vi "UHR-Fleezers Control (host) - Lorentz v4.vi"() -> ()   [LabVIEW 2014] (continued)
        n116 = local read "Channel 1"() -> (w331:T28)
        n117 = Array To Cluster(array=w333) -> (cluster=w332:T42)
        n118 = local read "Channel 3"() -> (w329:T28)
        n119 = Unbundle(w332) -> ("[0]"=w326:sgl, "[1]"=w325:sgl, "[2]"=w324:sgl, "[3]"=w323:sgl, "[4]"=w322:sgl, "[5]"=w321:sgl, "[6]"=w320:sgl, "[7]"=w319:sgl, "[8]"=w318:sgl, "[9]"=w317:sgl, "[10]"=w316:sgl, "[11]"=w315:sgl, "[12]"=w314:sgl, "[13]"=w313:sgl, "[14]"=w312:sgl)
        n120 = Bundle By Name(cluster=w331, "X Pos (mm)"=w326, "Y Pos (mm)"=w325, "Z Pos (mm)"=w324) -> (w311:T28)
        n121 = Bundle By Name(cluster=w330, "X Pos (mm)"=w323, "Y Pos (mm)"=w322, "Z Pos (mm)"=w321) -> (w310:T28)
        n122 = Bundle By Name(cluster=w328, "X Pos (mm)"=w317, "Y Pos (mm)"=w316, "Z Pos (mm)"=w315) -> (w308:T28)
        n123 = Bundle By Name(cluster=w329, "X Pos (mm)"=w320, "Y Pos (mm)"=w319, "Z Pos (mm)"=w318) -> (w309:T28)
        n124 = Bundle By Name(cluster=w327, "X Pos (mm)"=w314, "Y Pos (mm)"=w313, "Z Pos (mm)"=w312) -> (w307:T28)
        n125 = property on="Channel 2" class="Clust (strict)"("Value"=w310) -> ()  [unwired: 2 in, 2 out]
        n126 = property on="Channel 5" class="Clust (strict)"("Value"=w307) -> ()  [unwired: 2 in, 2 out]
        n127 = property on="Channel 1" class="Clust (strict)"("Value"=w311) -> ()  [unwired: 2 in, 2 out]
        n128 = property on="Channel 3" class="Clust (strict)"("Value"=w309) -> ()  [unwired: 2 in, 2 out]
        n129 = property on="Channel 4" class="Clust (strict)"("Value"=w308) -> ()  [unwired: 2 in, 2 out]
      }
    }
    n130 = Merge Errors(w100, w99, w98) -> (w97:errorcluster)
    n131 = property on="Motor Error Cluster out" class="Clust (strict)"("Val(Sgnl)"=w97) -> ()  [unwired: 2 in, 2 out]
  }
  n132 = disable-structure shown="Disabled" {
    frame Disabled {
      w347 = T34 0 items=["Grayscale (U8)", "Grayscale (I16)", "Grayscale (SGL)", "Complex (CSG)", "RGB (U32)", "HSL (U32)", "RGB (U64)", "Grayscale (U16)"] ("Image Type")
      n133 = call <vilib>:"IMAQdx Open Camera.vi"("Session In"=T43 "cam0") -> ("error out"=w351:errorcluster, "Session Out"=w350:T43)  [unwired: 9 in]
      n134 = call <vilib>:"IMAQdx Configure Grab.vi"("error in"=w351, "Session In"=w350) -> ("error out"=w342:errorcluster, "Session Out"=w349:T43)  [unwired: 8 in]
      n135 = call "IMAQ Create"("Image Name"="untitled", "Image Type"=w347) -> ("New Image"=w353:T1)  [unwired: 3 in, 1 out]
      n136 = while {
        tunnel: w353 -> [w359]
        tunnel: w349 -> [w360]
        tunnel: w342 -> [w358]
        tunnel: [w356] -> w346
        tunnel: [w357] -> w345
        tunnel: [w355] -> w343
        stop <- w354 stop-if-true
        n137 = call <vilib>:"IMAQdx Grab.vi"("error in"=w358, "Image In"=w359, "Session In"=w360) -> ("error out"=w356:errorcluster, "Image Out"=w355:T1, "Session Out"=w357:T43)  [unwired: 5 in, 1 out]
        "Image" <- w355
        n138 = local read "Stop All"() -> (w354:bool)
      }
      n139 = call <vilib>:"IMAQdx Close Camera.vi"("error in"=w346, "Session In"=w345) -> ("error out"=→"error out 4":errorcluster)  [unwired: 9 in]
      n140 = call "IMAQ Dispose"("Image"=w343) -> ()  [unwired: 5 in, 1 out]
    }
    frame Enabled {
    }
  }
  n141 = for {
    tunnel: w14 -> [w363] mode=indexing
    tunnel: w7 -> [w362] mode=indexing
    tunnel: [w361] -> w15 mode=indexing
    n142 = call "TLMotorStopCtrl.vi"("Error In (No Error)"=w362, "Motor Ref"=w363) -> ("Error Out"=w361:errorcluster)  [unwired: 4 in, 1 out]
  }
  n143 = call-poly <vilib>:"Close Input Device.vi"("error in (no error)"=w9, "device ID"=w8) -> ("error out"=w6:errorcluster)  [unwired: 8 in]
  n144 = Merge Errors(w15, w5, w6, w1) -> (→"Motor Error Cluster out":errorcluster)
  n145 = disable-structure shown="Enabled" {
    frame Enabled {
      w390 = FALSE
      # "This Control added by\nRonen to enable direct\nControl of pressure pulse\nlength to enable fine flow\ncontrol"
      # "Start out with all lines set to zero"
      n146 = Format Into String(format string="%s/port0/line5:1, %s/port1/line0:3", "DAQmx Device Name", "DAQmx Device Name") -> (resulting string=w382:string)  [unwired: 2 in, 1 out]
      n147 = Format Into String(format string="%s/ai0", "DAQmx Device Name") -> (resulting string=w380:string)  [unwired: 2 in, 1 out]
      n148 = In Range and Coerce(upper limit=100.0, x="Pulse Duration (0-100 ms)", lower limit=0.0) -> (coerced(x)=w365:dbl)  [unwired: 1 out]
      n149 = Bundle By Name(cluster=T44 {"daqmx_channel"="", "terminal_configuration"=""} ("Pressure Control Config"), "daqmx_channel"=w380, "terminal_configuration"="RSE") -> (w397:T44)
      n150 = To Unsigned Long Integer(number=w365) -> (unsigned 32bit integer=w364:u32)
      n151 = Bundle("Pressure up", "TTL line # Pressure Up"=u8 6, w390, w390) -> (w388:T45)  [unwired: 1 in]
      n152 = Bundle("Pressure down", "TTL line # Pressure Down"=u8 8, w390, w390) -> (w389:T46)  [unwired: 1 in]
      n153 = Bundle("Pressure vacuum", "TTL line # Pressure Vacuum"=u8 7, w390, w390) -> (w387:T47)  [unwired: 1 in]
      n154 = Build Array(w388, w389, w387) -> (w386:T48)
      n155 = call "Initialize.vi"("Pulse duration (ms)"=w364, "TTL Ports"=w382, "TTL in"=refnum<class "TTL.lvclass"> refnum ("TTL.lvclass")) -> ("error out"=w385:errorcluster, "TTL out"=w374:refnum<class "TTL.lvclass">)  [unwired: 7 in]
      n156 = call "Initialize.vi"("TTL Lines"=w386, "error in (no error)"=w385, "TTL"=w374, "Pressure Control Config"=w397, "Pressure Control in"=refnum<class "Pressure Control.lvclass"> refnum ("Pressure Control.lvclass")) -> ("error out"=w402:errorcluster, "Pressure Control out"=w384:refnum<class "Pressure Control.lvclass">)  [unwired: 5 in]
      n157 = call "Get line states.vi"("error in (no error)"=w402, "TTL in"=w374) -> ("error out"=w369:errorcluster, "Current line states"=w370:bool[], "TTL out"=w373:refnum<class "TTL.lvclass">)  [unwired: 7 in]
      n158 = Array Size(array=w370) -> (size(s)=w371:i32)
      n159 = for {
        N: w371 -> [_]
        shift-right: [w408] -> w372
        shift-left: w373 -> [w409]
        shift-right: [w406] -> w403
        shift-left: w369 -> [w407]
        i -> [w405]
        n160 = call "Set line.vi"("error in (no error)"=w407, "Action"=enum16{"Open", "Close", "Toggle"}."Open", "Line number"=w405, "TTL in"=w409) -> ("error out"=w406:errorcluster, "TTL out"=w408:refnum<class "TTL.lvclass">)  [unwired: 6 in]
      }
      n161 = case shown="No Error" w403 {
        selector: w403 -> [_ w463]
        tunnel: w384 -> [w414 _]
        tunnel: w372 -> [w413 _]
        tunnel: [w410 w462] -> w377
        frame No Error {
          n162 = while {
            shift-right: [w422] -> w411
            shift-left: w414 -> [w421]
            shift-right: [w420] -> w412
            shift-left: w413 -> [w419]
            stop <- w417 stop-if-true
            n163 = call "Get pressure.vi"("Pressure Control in"=w421) -> ("Pressure"=→"Pressure":dbl)  [unwired: 7 in, 3 out]
            n164 = event shown="[7] \"Pulse Duration (0-100 ms)\": Value Change" {
              selector: _ -> [_ _ _ _ _ _ _ _]
              dyn-events: _ -> [_ _ _ _ _ _ _ _]
              timeout: 100 -> [_ _ _ _ _ _ _ _]
              tunnel: [w425 w428 w429 w434 w438 w443 w448 w460] -> w422
              tunnel: w421 -> [w425 w428 w430 w435 w439 w444 w449 w461]
              tunnel: [w424 w427 w431 w436 w440 w445 w450 w458] -> w420
              tunnel: w419 -> [w424 w427 w431 w436 w440 w445 w450 w459]
              tunnel: [_ TRUE _ _ _ _ _ _] -> w417
              tunnel: [_ _ w432 w437 w441 w446 w451 w457] -> w416
              event Timeout {
                n165 = event-data() -> ()  [unwired: 1 in, 2 out]
              }
              event "Stop All": Value Change {
                n166 = event-data() -> ()  [unwired: 1 in, 6 out]
              }
              event "Vent pressure": Value Change {
                n167 = event-data() -> ()  [unwired: 1 in, 5 out]
                n168 = call "Vent.vi"("Pressure Control in"=w430) -> ("error out"=w432:errorcluster, "Pressure Control out"=w429:refnum<class "Pressure Control.lvclass">)  [unwired: 9 in]
              }
              event "Vacuum": Value Change {
                n169 = event-data() -> ("NewVal"=w433:bool)  [unwired: 1 in, 4 out]
                n170 = call "Set vacuum.vi"("Vacuum?"=w433, "Pressure Control in"=w435) -> ("error out"=w437:errorcluster, "Pressure Control out"=w434:refnum<class "Pressure Control.lvclass">)  [unwired: 8 in]
              }
              event "Set zero pressure": Value Change {
                n171 = event-data() -> ()  [unwired: 1 in, 5 out]
                n172 = call "Set zero pressure to current pressure.vi"("Pressure Control in"=w439) -> ("error out"=w441:errorcluster, "Pressure Control out"=w438:refnum<class "Pressure Control.lvclass">)  [unwired: 8 in, 1 out]
              }
              event "Pressure Up": Value Change {
                n173 = event-data() -> ()  [unwired: 1 in, 5 out]
                n174 = call "Pressure pulse.vi"("Up or down?"=enum16{"Up", "Down"}."Up", "Pressure Control in"=w444) -> ("error out"=w446:errorcluster, "Pressure Control out"=w443:refnum<class "Pressure Control.lvclass">)  [unwired: 8 in]
              }
              event "Pressure Down": Value Change {
                n175 = event-data() -> ()  [unwired: 1 in, 5 out]
                n176 = call "Pressure pulse.vi"("Up or down?"=enum16{"Up", "Down"}."Down", "Pressure Control in"=w449) -> ("error out"=w451:errorcluster, "Pressure Control out"=w448:refnum<class "Pressure Control.lvclass">)  [unwired: 8 in]
              }
              event "Pulse Duration (0-100 ms)": Value Change {
                # "Event added by Ronen to allow for changes\nin pulse duration as program is running"
                n177 = event-data() -> ()  [unwired: 1 in, 6 out]
                n178 = local read "Pulse Duration (0-100 ms)"() -> (w455:dbl)
                n179 = In Range and Coerce(upper limit=100.0, x=w455, lower limit=0.0) -> (coerced(x)=w453:dbl)  [unwired: 1 out]
                n180 = To Unsigned Long Integer(number=w453) -> (unsigned 32bit integer=w452:u32)
                n181 = call "Change TTL - Ronen.vi"("Pulse Duration (ms)"=w452, "TTL.lvclass"=w459) -> ("error out"=w457:errorcluster, "TTL.lvclass"=w458:refnum<class "TTL.lvclass">)  [unwired: 8 in]
                n182 = call "Update TTL - Ronen.vi"("TTL.lvclass"=w458, "Pressure Control in"=w461) -> ("Pressure Control out"=w460:refnum<class "Pressure Control.lvclass">)  [unwired: 8 in, 1 out]
              }
            }
            n183 = call <vilib>:"Simple Error Handler.vi"("error in (no error)"=w416) -> ()  [unwired: 4 in, 5 out]
          }
          n184 = call "Close.vi"("Pressure Control in"=w411) -> ("error out"=w415:errorcluster)  [unwired: 9 in, 1 out]
          n185 = call "Close.vi"("error in (no error)"=w415, "TTL in"=w412) -> ("error out"=w410:errorcluster)  [unwired: 8 in, 1 out]
        }
        frame Error {
          n186 = call <vilib>:"Simple Error Handler.vi"("error in (no error)"=w463) -> ("error out"=w462:errorcluster)  [unwired: 4 in, 4 out]
        }
      }
      n187 = property on="DAQmx Device Name" class="DAQmxName"("Visible"=FALSE) -> ()  [unwired: 2 in, 2 out]
      n188 = call <vilib>:"Clear Errors.vi"("error in (no error)"=w377) -> ("error out"=w375:errorcluster)  [unwired: 5 in, 1 out]
      n189 = property on="DAQmx Device Name" class="DAQmxName"(error in=w375, "Visible"=TRUE) -> ()  [unwired: 1 in, 2 out]
    }
    frame Disabled {
    }
  }
  n190 = disable-structure shown="Disabled" {
    disable-tunnel: [w495 _] -> w76
    disable-tunnel: [w492 _] -> w65
    disable-tunnel: [w491 _] -> w64
    disable-tunnel: [w486 _] -> w60
    disable-tunnel: [w485 _] -> w59
    disable-tunnel: [w484 _] -> w58
    disable-tunnel: [w483 _] -> w57
    disable-tunnel: [w480 _] -> w49
    disable-tunnel: [w475 _] -> w30
    disable-tunnel: [w468 _] -> w29
    disable-tunnel: [w465 _] -> w28
    frame Disabled {
      w467 = u16 20 items=["1.0"=10, "1.5"=15, "2.0"=20] ("stop bits (10: 1 bit)")
      w478 = u16 20 items=["1.0"=10, "1.5"=15, "2.0"=20] ("stop bits (10: 1 bit)")
      w481 = u16 10 items=["1.0"=10, "1.5"=15, "2.0"=20] ("stop bits (10: 1 bit)")
      w487 = u16 20 items=["1.0"=10, "1.5"=15, "2.0"=20] ("stop bits (10: 1 bit)")
      w489 = u16 20 items=["1.0"=10, "1.5"=15, "2.0"=20] ("stop bits (10: 1 bit)")
      w493 = u16 20 items=["1.0"=10, "1.5"=15, "2.0"=20] ("stop bits (10: 1 bit)")
      # "Bottom 1 Harvard"
      # "Top 3 Harvard"
      # "Center Harvard"
      n191 = call-poly "VISA Configure Serial Port"("VISA resource name"=refnum<visa-resource-name> "COM2", "baud rate (9600)"=u32 9600, "stop bits (10: 1 bit)"=w478) -> ("VISA resource name out"=w468:refnum<visa-resource-name>, "error out"=→"Preamp Error Out":errorcluster)  [unwired: 4 in, 7 out]
      n192 = call-poly "VISA Configure Serial Port"("VISA resource name"=refnum<visa-resource-name> "COM2", "baud rate (9600)"=u32 9600, "stop bits (10: 1 bit)"=w467) -> ("VISA resource name out"=w465:refnum<visa-resource-name>)  [unwired: 4 in, 8 out]
      n193 = call-poly "VISA Configure Serial Port"("VISA resource name"=refnum<visa-resource-name> "COM7", "baud rate (9600)"=u32 115200, "stop bits (10: 1 bit)"=w481) -> ("VISA resource name out"=w480:refnum<visa-resource-name>, "error out"=w479:errorcluster)  [unwired: 4 in, 7 out]
      n194 = call-poly "VISA Configure Serial Port"("VISA resource name"=refnum<visa-resource-name> "COM5", "baud rate (9600)"=u32 115200, "stop bits (10: 1 bit)"=w487) -> ("VISA resource name out"=w484:refnum<visa-resource-name>, "error out"=w483:errorcluster)  [unwired: 4 in, 7 out]
      n195 = call-poly "VISA Configure Serial Port"("VISA resource name"=refnum<visa-resource-name> "COM4", "baud rate (9600)"=u32 115200, "stop bits (10: 1 bit)"=w489) -> ("VISA resource name out"=w486:refnum<visa-resource-name>, "error out"=w485:errorcluster)  [unwired: 4 in, 7 out]
      n196 = call-poly "VISA Configure Serial Port"("VISA resource name"=refnum<visa-resource-name> "COM6", "baud rate (9600)"=u32 115200, "stop bits (10: 1 bit)"=w493) -> ("VISA resource name out"=w491:refnum<visa-resource-name>, "error out"=w492:errorcluster)  [unwired: 4 in, 7 out]
      n197 = call-poly "VISA Configure Serial Port"("VISA resource name"=refnum<visa-resource-name> "COM1") -> ("VISA resource name out"=w475:refnum<visa-resource-name>, "error out"=w495:errorcluster)  [unwired: 5 in, 8 out]
      "Stage Control Serial Error" <- w495
      n198 = local write "Blue Error Out"(w479) -> ()
    }
    frame Enabled {
    }
  }
  n199 = call "IMAQ Create"("Image Name"="APD 1 Image", "Image Type"=w53) -> ("New Image"=w70:T1)  [unwired: 3 in, 1 out]
  n200 = call "IMAQ Create"("Image Name"="APD 2 Image", "Image Type"=w53) -> ("New Image"=w69:T1)  [unwired: 3 in, 1 out]
  n201 = call "IMAQ Create"("Image Name"="APD 3 Image", "Image Type"=w53) -> ("New Image"=w52:T1)  [unwired: 3 in, 1 out]
  n202 = call "IMAQ Create"("Image Name"="Det. X Image", "Image Type"=w53) -> ("New Image"=w68:T1)  [unwired: 3 in, 1 out]
  n203 = call "IMAQ Create"("Image Name"="Det. Y Image", "Image Type"=w53) -> ("New Image"=w67:T1)  [unwired: 3 in, 1 out]
  n204 = Bundle("New Image"=w70, "New Image"=w69, "New Image"=w52, "New Image"=w68, "New Image"=w67) -> (w66:T49)  [unwired: 1 in]
  n205 = xnode "Open FPGA VI Reference"("resource name"=T33 "RIO0") -> ("FPGA VI Reference Out"=w47:T50, "error out"=w46:errorcluster)  [unwired: 1 in]
  n206 = xnode "Invoke Method"("FPGA VI Reference In"=w47, "error in"=w46) -> ("FPGA VI Reference Out"=w27:T50, "error out"=→"FPGA error out":errorcluster)
  n207 = Subtract(x=w25, y="Maximum Delta\n(MHz)") -> (x-y=w23:dbl)
  n208 = Bundle By Name(cluster=T24 {"Minimum"=60.0, "Maximum"=90.0, "Increment"=1.0} ("Min Max Inc"), "Minimum"=w23, "Maximum"=w25) -> (w22:T24)
  n209 = node-c288() -> (w73:T35)  [unwired: 4 in]
  n210 = timed-loop "Run Scripts, including: stage motion" {
    tunnel: w76 -> [w506]
    tunnel: w30 -> [w507]
    tunnel: [w507] -> w75
    tunnel: [w506] -> w74
    timing: w73 -> [_]
    timing-out: [_] -> w72
    tunnel: w64 -> [w505]
    tunnel: w65 -> [w504]
    tunnel: w60 -> [w501]
    tunnel: w59 -> [w500]
    tunnel: w58 -> [w502]
    tunnel: w57 -> [w503]
    tunnel: w49 -> [w499]
    tunnel: w42 -> [w498]
    tunnel: w29 -> [w497]
    tunnel: w28 -> [w496]
    stop <- w508 stop-if-true
    n211 = node-c288() -> ()  [unwired: 1 in, 1 out]
    n212 = event shown="[17] \"Got Bead 1\": Value Change" {
      selector: _ -> [_ _ _ _ _ _ _ _ _ _ _ _ _ _ _ _ _ _ _ _ _ _ _ _ _ _ _ _]
      dyn-events: _ -> [_ _ _ _ _ _ _ _ _ _ _ _ _ _ _ _ _ _ _ _ _ _ _ _ _ _ _ _]
      timeout: _ -> [_ _ _ _ _ _ _ _ _ _ _ _ _ _ _ _ _ _ _ _ _ _ _ _ _ _ _ _]
      tunnel: ["Set Position" "Move to Position" _ _ _ _ _ _ "Read Harvard" _ _ _ _ _ _ _ _ "Got Bead 1" "Force FB Data\nScript" _ "Got Bead 2" _ "Take Stepping Data" _ "Take Detection Laser\nImage" _ _ _] -> _
      tunnel: [_ _ _ _ _ _ _ _ _ _ _ _ _ _ _ _ _ _ _ _ _ _ _ _ _ _ w1435 _] -> w508
      tunnel: w506 -> [w527 w535 w548 w578 _ _ _ _ _ w715 w749 w775 w807 w896 w925 w1057 w1084 _ w1126 _ _ _ _ _ _ _ _ _]
      tunnel: w507 -> [w528 w536 w549 w579 _ _ _ _ _ w716 w750 w776 w808 w897 w926 w1058 w1085 _ w1127 _ _ _ _ _ _ _ _ _]
      tunnel: w505 -> [_ _ _ _ _ _ _ _ w700 _ _ _ _ _ _ _ _ _ _ _ _ _ _ _ _ _ _ _]
      tunnel: w504 -> [_ _ _ _ _ _ _ _ w699 _ _ _ _ _ _ _ _ _ _ _ _ _ _ _ _ _ _ _]
      tunnel: w503 -> [_ _ _ _ _ _ _ _ _ _ _ _ _ _ _ _ _ _ _ _ _ _ _ _ _ _ _ _]
      tunnel: w502 -> [_ _ _ _ _ _ _ _ _ _ _ _ _ _ _ _ _ _ _ _ _ _ _ _ _ _ _ _]
      tunnel: w501 -> [_ _ _ _ _ _ _ _ _ _ _ _ _ _ _ _ _ _ _ _ _ _ _ _ _ _ _ _]
      tunnel: w500 -> [_ _ _ _ _ _ _ _ _ _ _ _ _ _ _ _ _ _ _ _ _ _ _ _ _ _ _ _]
      tunnel: w499 -> [_ _ _ _ w606 w613 w641 w660 _ _ _ _ _ _ _ _ _ _ _ _ _ _ _ _ _ _ w1434 _]
      tunnel: w498 -> [_ _ _ _ _ _ _ _ _ _ _ _ _ _ _ _ _ _ _ _ _ _ _ _ _ w1301 _ _]
      tunnel: w497 -> [_ _ _ _ _ _ _ _ _ _ _ _ _ _ _ _ _ _ _ _ _ _ _ _ _ _ _ w1445]
      tunnel: w496 -> [_ _ _ _ _ _ _ _ _ _ _ _ _ _ _ _ _ _ _ _ _ _ _ _ _ _ _ w1440]
      tunnel: [_ _ _ _ _ _ _ _ _ _ _ _ _ _ _ _ _ _ _ _ _ "Get New Beads" _ _ _ _ _ _] -> _
      event "Set Position", "Set Position 2", "Set Position 3", "Set Position 4", "Set Position 5", "Set Position 1", "Set Position 6": Value Change {
        n213 = event-data() -> ()  [unwired: 1 in, 5 out]
        n214 = Build Array("Set Position 1", "Set Position 2", "Set Position 3", "Set Position 4", "Set Position 5", "Set Position 6") -> (w526:bool[])
        n215 = Boolean Array To Number(Boolean array=w526) -> (number=w525:u32)
        n216 = Logarithm Base 2(1:w525) -> (0:w517:dbl)
        n217 = call "Read Stage Position.vi"("error in"=w527, "VISA resource name in"=w528) -> ("Current Position"=w532:cluster{dbl, dbl, dbl}, "error out"=w531:errorcluster)  [unwired: 2 out]
        n218 = Decrement(x="Position") -> (x-1=w515:dbl)
        n219 = Greater Or Equal?(x=w517, y=0.0) -> (x >= y?=w518:bool)
        n220 = Cluster To Array(cluster=w532) -> (array=w529:dbl[])
        n221 = local write "Stage Control Serial Error"(w531) -> ()
        n222 = Select(t=w517, s=w518, f=w515) -> (s? t:f=w514:dbl)
        n223 = Increment(x=w514) -> (x+1=w513:dbl)
        n224 = Build Array (concatenate)(w513, w529) -> (w512:dbl[])
        n225 = Replace Array Subset(array="Saved Stage Positions", new element=w512, index (row)=w514) -> (w530:dbl[][])  [unwired: 1 in]
        n226 = local write "Saved Stage Positions"(w530) -> ()
      }
      event "Move to Position": Value Change {
        n227 = event-data() -> ()  [unwired: 1 in, 5 out]
        n228 = flat-sequence {
          tunnel: w536 -> [w540]
          tunnel: w535 -> [w539]
          frame #0 {
            n229 = local read "Saved Stage Positions"() -> (w542:dbl[][])
            n230 = local read "Position"() -> (w541:dbl)
            n231 = local write "Stage Moving"(TRUE ("Stage Moving")) -> ()
            n232 = call "move to saved stage position.vi"("error in"=w539, "Stage VISA resource name in"=w540, "Position"=w541, "Saved Stage Positions"=w542) -> ("error out"=w538:errorcluster)  [unwired: 1 out]
            n233 = local write "Stage Control Serial Error"(w538) -> ()
          }
          frame #1 {
            n234 = call <vilib>:"Beep.vi"() -> ()  [unwired: 3 in, 9 out]
            n235 = local write "Stage Moving"(FALSE ("Stage Moving")) -> ()
          }
        }
      }
      event "Move Cap. 1 (DNA Bottom)": Value Change {
        n236 = event-data() -> ()  [unwired: 1 in, 5 out]
        n237 = local write "Move Cap. 1 (DNA Bottom)"(FALSE ("Move Cap. 1 (DNA Right)")) -> ()
        n238 = flat-sequence {
          tunnel: w548 -> [w551]
          tunnel: w549 -> [w552]
          tunnel: [w552] -> w546
          tunnel: [w551] -> w545
          tunnel: w546 -> [w554]
          tunnel: w545 -> [w553]
          frame #0 {
            n239 = property on="Sample Channel\nFlow" class="Bool (strict)"("Val(Sgnl)"="Cap 1 Samp Flow ON") -> ()  [unwired: 2 in, 2 out]
          }
          frame #1 {
            n240 = local read "Saved Stage Positions"() -> (w564:dbl[][])
            n241 = local write "Stage Moving"(TRUE ("Stage Moving")) -> ()
            n242 = Array Subset(array=w564, index (row)=0 ("index"), length (row)=1 ("length"), index (col)=1 ("index"), length (col)=3 ("length")) -> (w561:dbl[][])
            n243 = Reshape Array(w561, 3 ("dimension size")) -> (w559:dbl[])
            n244 = Array To Cluster(array=w559) -> (cluster=w558:cluster{"[0]":dbl, "[1]":dbl, "[2]":dbl})
            n245 = call "Set Stage Position.vi"("Position"=w558, "error in"=w553, "VISA resource name in"=w554) -> ("error out"=w557:errorcluster)  [unwired: 2 out]
            n246 = local write "Stage Control Serial Error"(w557) -> ()
          }
          frame #2 {
            n247 = local write "Stage Moving"(FALSE ("Stage Moving")) -> ()
            n248 = case shown="True" "Cap 1 Flow ON" {
              frame False {
              }
              frame True {
                n249 = property on="Inject Pump 1" class="Bool (strict)"("Val(Sgnl)"=TRUE ("Value (Signaling)")) -> ()  [unwired: 2 in, 2 out]
              }
            }
            n250 = call <vilib>:"Beep.vi"() -> ()  [unwired: 3 in, 9 out]
          }
          frame #3 {
            n251 = property on="Sample Channel\nFlow" class="Bool (strict)"("Val(Sgnl)"=FALSE ("Value (Signaling)")) -> ()  [unwired: 2 in, 2 out]
            n252 = local read "Cap. 2 BD T1?\n(ADig T1, DNA T2)"() -> (w571:bool)
            n253 = case shown="True" w571 {
              tunnel: "Cap 1 T ON" -> [w573 w574]
              frame False {
                n254 = property on="Trap 1 (ON/OFF)" class="Bool (strict)"("Val(Sgnl)"=w573) -> ()  [unwired: 2 in, 2 out]
              }
              frame True {
                n255 = property on="Trap 2 (ON/OFF)" class="Bool (strict)"("Val(Sgnl)"=w574) -> ()  [unwired: 2 in, 2 out]
              }
            }
            n256 = property on="Got Bead 2" class="Bool"("Key Focus"=TRUE) -> ()  [unwired: 2 in, 2 out]
          }
        }
      }
      event "Move Cap. 2 (ADig Top)": Value Change {
        n257 = event-data() -> ()  [unwired: 1 in, 5 out]
        n258 = local write "Move Cap. 2 (ADig Top)"(FALSE ("Move Cap. 2 (ADig Left)")) -> ()
        n259 = flat-sequence {
          tunnel: w578 -> [w581]
          tunnel: w579 -> [w582]
          tunnel: [w582] -> w576
          tunnel: [w581] -> w575
          tunnel: w576 -> [w585]
          tunnel: w575 -> [w584]
          frame #0 {
            n260 = property on="Sample Channel\nFlow" class="Bool (strict)"("Val(Sgnl)"="Cap 2 Samp Flow ON") -> ()  [unwired: 2 in, 2 out]
          }
          frame #1 {
            w583 = FALSE ("Value (Signaling)")
            n261 = local read "Saved Stage Positions"() -> (w595:dbl[][])
            n262 = local write "Stage Moving"(TRUE ("Stage Moving")) -> ()
            n263 = Array Subset(array=w595, index (row)=1 ("index"), length (row)=1 ("length"), index (col)=1 ("index"), length (col)=3 ("length")) -> (w592:dbl[][])
            n264 = Reshape Array(w592, 3 ("dimension size")) -> (w590:dbl[])
            n265 = property on="Trap 1 (ON/OFF)" class="Bool (strict)"("Val(Sgnl)"=w583) -> ()  [unwired: 2 in, 2 out]
            n266 = property on="Trap 1 (ON/OFF)" class="Bool (strict)"("Val(Sgnl)"=w583) -> ()  [unwired: 2 in, 2 out]
            n267 = Array To Cluster(array=w590) -> (cluster=w589:cluster{"[0]":dbl, "[1]":dbl, "[2]":dbl})
            n268 = call "Set Stage Position.vi"("Position"=w589, "error in"=w584, "VISA resource name in"=w585) -> ("error out"=w588:errorcluster)  [unwired: 2 out]
            n269 = local write "Stage Control Serial Error"(w588) -> ()
          }
          frame #2 {
            n270 = local write "Stage Moving"(FALSE ("Stage Moving")) -> ()
            n271 = call <vilib>:"Beep.vi"() -> ()  [unwired: 3 in, 9 out]
            n272 = case shown="True" "Cap 2 Flow ON" {
              frame False {
              }
              frame True {
                n273 = property on="Inject Pump 3" class="Bool (strict)"("Val(Sgnl)"=TRUE ("Value (Signaling)")) -> ()  [unwired: 2 in, 2 out]
              }
            }
          }
          frame #3 {
            n274 = property on="Sample Channel\nFlow" class="Bool (strict)"("Val(Sgnl)"=FALSE ("Value (Signaling)")) -> ()  [unwired: 2 in, 2 out]
            n275 = case shown="False" "Cap. 2 BD T1?\n(ADig T1, DNA T2)" {
              tunnel: "Cap 2 T ON" -> [w604 w605]
              frame False {
                n276 = property on="Trap 2 (ON/OFF)" class="Bool (strict)"("Val(Sgnl)"=w604) -> ()  [unwired: 2 in, 2 out]
              }
              frame True {
                n277 = property on="Trap 1 (ON/OFF)" class="Bool (strict)"("Val(Sgnl)"=w605) -> ()  [unwired: 2 in, 2 out]
              }
            }
            n278 = property on="Got Bead 1" class="Bool"("Key Focus"=TRUE) -> ()  [unwired: 2 in, 2 out]
          }
        }
      }
      event "Send string\nto Blue Laser": Value Change {
        n279 = event-data() -> ()  [unwired: 1 in, 5 out]
        n280 = flat-sequence {
          tunnel: w606 -> [w607]
          frame #0 {
            n281 = call "serial write macro.vi"("String"="command string", "Delay (ms)"="Delay (ms)", "VISA resource name"=w607) -> ("read buffer"=→"read blue buffer":string, "error out"=→"Blue Error Out":errorcluster)  [unwired: 1 out]
            "command string sent" <- "command string"
          }
          frame #1 {
            n282 = local write "Send string\nto Blue Laser"(FALSE ("Send string")) -> ()
          }
        }
      }
      event "Get Blue Laser State": Value Change {
        n283 = event-data() -> ()  [unwired: 1 in, 5 out]
        n284 = local read "Delay (ms)"() -> (w614:i32)
        n285 = flat-sequence {
          tunnel: w614 -> [w622]
          tunnel: w613 -> [w625]
          tunnel: [w623] -> w618
          tunnel: [w622] -> w617
          tunnel: [w632] -> w616
          tunnel: [w629] -> w615
          tunnel: w618 -> [w630]
          tunnel: w617 -> [w629]
          tunnel: w616 -> [w638]
          tunnel: w615 -> [w636]
          frame #0 {
            w620 = "l?"
            n286 = local write "command string sent"(w620) -> ()
            n287 = call "serial write macro.vi"("String"=w620, "Delay (ms)"=w622, "VISA resource name"=w625) -> ("read buffer"=w621:string, "VISA resource name out"=w623:refnum<visa-resource-name>)  [unwired: 1 out]
            n288 = Decimal String To Number(string=w621) -> (number=w624:i32)  [unwired: 2 in, 1 out]
            n289 = Not Equal To 0?(x=w624) -> (x != 0?=→"Laser On":bool)
            n290 = local write "read blue buffer"(w621) -> ()
          }
          frame #1 {
            w627 = "games?" ("String")
            n291 = local write "command string sent"(w627) -> ()
            n292 = call "serial write macro.vi"("String"=w627, "Delay (ms)"=w629, "VISA resource name"=w630) -> ("read buffer"=w628:string, "VISA resource name out"=w632:refnum<visa-resource-name>)  [unwired: 1 out]
            n293 = Decimal String To Number(string=w628) -> (number=w631:i32)  [unwired: 2 in, 1 out]
            n294 = local write "read blue buffer"(w628) -> ()
            n295 = Not Equal To 0?(x=w631) -> (x != 0?=→"Analog Modulation":bool)
          }
          frame #2 {
            w634 = "gdmes?" ("String")
            n296 = local write "command string sent"(w634) -> ()
            n297 = call "serial write macro.vi"("String"=w634, "Delay (ms)"=w636, "VISA resource name"=w638) -> ("read buffer"=w635:string)  [unwired: 2 out]
            n298 = Decimal String To Number(string=w635) -> (number=w637:i32)  [unwired: 2 in, 1 out]
            n299 = Not Equal To 0?(x=w637) -> (x != 0?=→"Digital Modulation":bool)
            n300 = local write "read blue buffer"(w635) -> ()
          }
          frame #3 {
            n301 = local write "Get Blue Laser State"(FALSE) -> ()
          }
        }
      }
      event "Blue Laser Power (mW)\n(Constant Power Mode)", "Blue Laser Modulation\nPower (mW)": Value Change {
        n302 = event-data() -> ()  [unwired: 1 in, 5 out]
        n303 = flat-sequence {
          tunnel: w641 -> [w647]
          tunnel: [w645] -> w640
          tunnel: w640 -> [w654]
          frame #0 {
            n304 = local read "Delay (ms)"() -> (w646:i32)
            n305 = Concatenate Strings("slmp " ("string"), "Blue Laser Modulation\nPower (mW)") -> (w642:string)
            n306 = call "serial write macro.vi"("String"=w642, "Delay (ms)"=w646, "VISA resource name"=w647) -> ("read buffer"=w643:string, "error out"=w644:errorcluster, "VISA resource name out"=w645:refnum<visa-resource-name>)
            n307 = local write "command string sent"(w642) -> ()
            n308 = local write "read blue buffer"(w643) -> ()
            n309 = local write "Blue Error Out"(w644) -> ()
          }
          frame #1 {
            n310 = local read "Delay (ms)"() -> (w653:i32)
            n311 = Concatenate Strings("p " ("string"), "Blue Laser Power (mW)\n(Constant Power Mode)") -> (w650:string)
            n312 = call "serial write macro.vi"("String"=w650, "Delay (ms)"=w653, "VISA resource name"=w654) -> ("read buffer"=w651:string, "error out"=w652:errorcluster)  [unwired: 1 out]
            n313 = local write "command string sent"(w650) -> ()
            n314 = local write "read blue buffer"(w651) -> ()
            n315 = local write "Blue Error Out"(w652) -> ()
          }
        }
      }
      event "Laser interlacing mode", "Blue Laser Modulation Mode", "Blue Laser ON": Value Change {
        n316 = event-data() -> ()  [unwired: 1 in, 5 out]
        n317 = flat-sequence {
          tunnel: w660 -> [w665]
          tunnel: [w664] -> w657
          tunnel: [w670] -> w659
          tunnel: w657 -> [w673]
          tunnel: w659 -> [w685]
          tunnel: [w679] -> w658
          tunnel: w658 -> [w692]
          frame #0 {
            n318 = local read "Blue Laser ON"() -> (w662:bool)
            n319 = local read "Delay (ms)"() -> (w663:i32)
            n320 = case shown="False" w662 {
              tunnel: ["l0" "l1"] -> w661
              frame False {
              }
              frame True {
              }
            }
            n321 = call "serial write macro.vi"("String"=w661, "Delay (ms)"=w663, "VISA resource name"=w665) -> ("error out"=w666:errorcluster, "VISA resource name out"=w664:refnum<visa-resource-name>)  [unwired: 1 out]
            n322 = local write "Blue Error Out"(w666) -> ()
          }
          frame #1 {
            n323 = local read "Laser interlacing mode"() -> (w675:enum32{"Laser ON", "Laser OFF", "Interlace"})
            n324 = case shown="\"Laser ON\"" w675 {
              tunnel: ["cp" "em" "l0"] -> w669
              frame "Laser ON" {
              }
              frame "Interlace" {
              }
              frame "Laser OFF", Default {
              }
            }
            n325 = local read "Delay (ms)"() -> (w674:i32)
            n326 = call "serial write macro.vi"("String"=w669, "Delay (ms)"=w674, "VISA resource name"=w673) -> ("read buffer"=w671:string, "error out"=w672:errorcluster, "VISA resource name out"=w670:refnum<visa-resource-name>)
            n327 = local write "command string sent"(w669) -> ()
            n328 = local write "read blue buffer"(w671) -> ()
            n329 = local write "Blue Error Out"(w672) -> ()
          }
          frame #2 {
            n330 = case shown="\"Analog Modulation\"" "Blue Laser Modulation Mode" {
              tunnel: ["sdmes 0" "sdmes 1" "sdmes 1"] -> w680
              frame "Analog Modulation" {
              }
              frame "Digital + Analog Modulation" {
              }
              frame "Digital Modulation", Default {
              }
            }
            n331 = local read "Delay (ms)"() -> (w683:i32)
            n332 = call "serial write macro.vi"("String"=w680, "Delay (ms)"=w683, "VISA resource name"=w685) -> ("read buffer"=w681:string, "error out"=w682:errorcluster, "VISA resource name out"=w679:refnum<visa-resource-name>)
            n333 = local write "command string sent"(w680) -> ()
            n334 = local write "read blue buffer"(w681) -> ()
            n335 = local write "Blue Error Out"(w682) -> ()
          }
          frame #3 {
            n336 = local read "Blue Laser Modulation Mode"() -> (w694:string)
            n337 = case shown="\"Digital Modulation\", Default" w694 {
              tunnel: ["sames 1" "sames 1" "sames 0"] -> w690
              frame "Analog Modulation" {
              }
              frame "Digital + Analog Modulation" {
              }
              frame "Digital Modulation", Default {
              }
            }
            n338 = local read "Delay (ms)"() -> (w693:i32)
            n339 = local write "command string sent"(w690) -> ()
            n340 = call "serial write macro.vi"("String"=w690, "Delay (ms)"=w693, "VISA resource name"=w692) -> ("read buffer"=w691:string, "error out"=w689:errorcluster)  [unwired: 1 out]
            n341 = local write "read blue buffer"(w691) -> ()
            n342 = local write "Blue Error Out"(w689) -> ()
          }
        }
      }
      event "Read Harvard": Value Change {
        n343 = event-data() -> ()  [unwired: 1 in, 5 out]
        n344 = Concatenate Strings("write buffer", "\r") -> (w702:string)
        n345 = VISA Write(VISA resource name=w700, write buffer=w702, error in (no error)=w699) -> (VISA resource name out=w711:refnum<visa-resource-name>, error out=w710:errorcluster)  [unwired: 1 out]
        n346 = stacked-sequence {
          tunnel: [w714] -> w709
          tunnel: w711 -> [w714]
          tunnel: w710 -> [w713]
          tunnel: [w713] -> w704
          frame #0 {
            n347 = Wait (ms)(milliseconds to wait=50) -> ()  [unwired: 1 out]
          }
        }
        n348 = property class="Instr"(reference=w709, error in=w704) -> (reference out=w708:refnum<visa-resource-name>, error out=w706:errorcluster, "Serial Settings:Number of Bytes at Serial Port"=w707:u32)
        "Serial Settings:Number of Bytes at Serial Port" <- w707
        n349 = VISA Read(VISA resource name=w708, byte count=w707, error in (no error)=w706) -> (read buffer=w705:string)  [unwired: 3 out]
        "read buffer" <- w705
        n350 = Fract/Exp String To Number(string=w705) -> ()  [unwired: 5 out]
      }
      event "+z", "-z": Value Change {
        n351 = event-data() -> ()  [unwired: 1 in, 5 out]
        n352 = flat-sequence {
          tunnel: w715 -> [w737]
          tunnel: w716 -> [w717]
          frame #0 {
            n353 = call "Read Stage Position.vi"("error in"=w737, "VISA resource name in"=w717) -> ("Current Position"=w722:cluster{dbl, dbl, dbl}, "error out"=w735:errorcluster, "VISA resource name out"=w736:refnum<visa-resource-name>)  [unwired: 1 out]
            n354 = local read "Saved Stage Positions"() -> (w746:dbl[][])
            n355 = Divide(x="z nudge increment (um)", y=1000.0) -> (x/y=w734:dbl)
            n356 = Boolean To (0,1)(Boolean="+z") -> (0, 1=w726:i16)
            n357 = Boolean To (0,1)(Boolean="-z") -> (0, 1=w727:i16)
            n358 = Array Subset(array=w746, index (row)=1 ("index"), length (row)=1 ("length"), index (col)=1 ("index"), length (col)=3 ("length")) -> (w743:dbl[][])
            n359 = Multiply(x=w726, y=w734) -> (x*y=w730:dbl)
            n360 = Multiply(x=w727, y=w734) -> (x*y=w728:dbl)
            n361 = Unbundle(w722) -> (w720:dbl, w719:dbl, w723:dbl)
            n362 = Negate(x=w728) -> (-x=w729:dbl)
            n363 = Reshape Array(w743, 3 ("dimension size")) -> (w741:dbl[])
            n364 = Add(x=w730, y=w729) -> (x+y=w731:dbl)
            n365 = Array To Cluster(array=w741) -> ()  [unwired: 1 out]
            n366 = Add(x=w731, y=w723) -> (x+y=w721:dbl)
            n367 = Bundle(cluster=w722, w720, w719, w721) -> (w718:cluster{dbl, dbl, dbl})
            n368 = call "Set Stage Position.vi"("Position"=w718, "error in"=w735, "VISA resource name in"=w736) -> ("error out"=w740:errorcluster)  [unwired: 2 out]
            n369 = local write "Stage Moving"(TRUE ("Stage Moving")) -> ()
            n370 = local write "Stage Control Serial Error"(w740) -> ()
          }
          frame #1 {
            n371 = local write "Stage Moving"(FALSE ("Stage Moving")) -> ()
          }
        }
      }
      event "-y", "+y": Value Change {
        n372 = event-data() -> ()  [unwired: 1 in, 5 out]
        n373 = flat-sequence {
          tunnel: w749 -> [w773]
          tunnel: w750 -> [w756]
          frame #0 {
            n374 = call "Read Stage Position.vi"("error in"=w773, "VISA resource name in"=w756) -> ("Current Position"=w759:cluster{dbl, dbl, dbl}, "error out"=w771:errorcluster, "VISA resource name out"=w772:refnum<visa-resource-name>)  [unwired: 1 out]
            n375 = Divide(x="y nudge increment (um", y=1000.0) -> (x/y=w770:dbl)
            n376 = Boolean To (0,1)(Boolean="+y") -> (0, 1=w762:i16)
            n377 = Boolean To (0,1)(Boolean="-y") -> (0, 1=w763:i16)
            n378 = Multiply(x=w762, y=w770) -> (x*y=w766:dbl)
            n379 = Multiply(x=w763, y=w770) -> (x*y=w764:dbl)
            n380 = Unbundle(w759) -> (w758:dbl, w753:dbl, w755:dbl)
            n381 = Negate(x=w764) -> (-x=w765:dbl)
            n382 = Add(x=w766, y=w765) -> (x+y=w767:dbl)
            n383 = Add(x=w767, y=w753) -> (x+y=w754:dbl)
            n384 = Bundle(cluster=w759, w758, w754, w755) -> (w757:cluster{dbl, dbl, dbl})
            n385 = call "Set Stage Position.vi"("Position"=w757, "error in"=w771, "VISA resource name in"=w772) -> ("error out"=w752:errorcluster)  [unwired: 2 out]
            n386 = local write "Stage Control Serial Error"(w752) -> ()
            n387 = local write "Stage Moving"(TRUE ("Stage Moving")) -> ()
          }
          frame #1 {
            n388 = local write "Stage Moving"(FALSE ("Stage Moving")) -> ()
          }
        }
      }
      event "-x", "+x": Value Change {
        n389 = event-data() -> ()  [unwired: 1 in, 5 out]
        n390 = flat-sequence {
          tunnel: w775 -> [w799]
          tunnel: w776 -> [w783]
          frame #0 {
            n391 = call "Read Stage Position.vi"("error in"=w799, "VISA resource name in"=w783) -> ("Current Position"=w785:cluster{dbl, dbl, dbl}, "error out"=w797:errorcluster, "VISA resource name out"=w798:refnum<visa-resource-name>)  [unwired: 1 out]
            n392 = Divide(x="x nudge increment (um)", y=1000.0) -> (x/y=w796:dbl)
            n393 = Boolean To (0,1)(Boolean="+x") -> (0, 1=w788:i16)
            n394 = Boolean To (0,1)(Boolean="-x") -> (0, 1=w789:i16)
            n395 = Multiply(x=w788, y=w796) -> (x*y=w792:dbl)
            n396 = Multiply(x=w789, y=w796) -> (x*y=w790:dbl)
            n397 = Unbundle(w785) -> (w777:dbl, w779:dbl, w782:dbl)
            n398 = Negate(x=w790) -> (-x=w791:dbl)
            n399 = Add(x=w792, y=w791) -> (x+y=w793:dbl)
            n400 = Add(x=w793, y=w777) -> (x+y=w778:dbl)
            n401 = Bundle(cluster=w785, w778, w779, w782) -> (w784:cluster{dbl, dbl, dbl})
            n402 = call "Set Stage Position.vi"("Position"=w784, "error in"=w797, "VISA resource name in"=w798) -> ("error out"=w780:errorcluster)  [unwired: 2 out]
            n403 = local write "Stage Control Serial Error"(w780) -> ()
            n404 = local write "Stage Moving"(TRUE ("Stage Moving")) -> ()
          }
          frame #1 {
            n405 = local write "Stage Moving"(FALSE ("Stage Moving")) -> ()
          }
        }
      }
      event "Cal/Data Acq. Spot": Value Change {
        # "Disabled by Ronen - we have our own way of controlling the location of calibration."
        n406 = event-data() -> ()  [unwired: 1 in, 5 out]
        n407 = flat-sequence {
          tunnel: w807 -> [w811]
          tunnel: w808 -> [w812]
          tunnel: [w812] -> w804
          tunnel: [w811] -> w803
          tunnel: w804 -> [w815]
          tunnel: w803 -> [w814]
          tunnel: ["Cal @ (MHz)"] -> w801
          tunnel: [w823] -> w805
          tunnel: w801 -> [w823]
          tunnel: w805 -> [w835]
          tunnel: ["W/ Offset 1"] -> w802
          tunnel: w805 -> [w856]
          tunnel: w802 -> [w854]
          frame #0 {
            n408 = property on="Sample Channel\nFlow" class="Bool (strict)"("Val(Sgnl)"="Daq spot flow on") -> ()  [unwired: 2 in, 2 out]
            n409 = Wait (ms)(milliseconds to wait=u32 250) -> ()  [unwired: 1 out]
          }
          frame #1 {
            n410 = disable-structure shown="Disabled" {
              disable-tunnel: w815 -> [w820 _]
              disable-tunnel: w814 -> [w819 _]
              frame Disabled {
                n411 = local read "Saved Stage Positions"() -> (w817:dbl[][])
                n412 = call "move to saved stage position.vi"("error in"=w819, "Stage VISA resource name in"=w820, "Position"="Cal Stage Position", "Saved Stage Positions"=w817) -> ("error out"=w818:errorcluster)  [unwired: 1 out]
                n413 = local write "Stage Control Serial Error"(w818) -> ()
              }
              frame Enabled {
              }
            }
            n414 = property on="Trap Delta (MHz)" class="DigNum (strict)"("Val(Sgnl)"="Cal @ (MHz)") -> ()  [unwired: 2 in, 2 out]
            n415 = local write "Stage Moving"(TRUE ("Stage Moving")) -> ()
          }
          frame #2 {
            n416 = local write "Stage Moving"(FALSE ("Stage Moving")) -> ()
            n417 = property on="Sample Channel\nFlow" class="Bool (strict)"("Val(Sgnl)"="Flow ON during cal?") -> ()  [unwired: 2 in, 2 out]
            n418 = call <vilib>:"Beep.vi"() -> ()  [unwired: 3 in, 9 out]
          }
          frame #3 {
            n419 = Wait (ms)(milliseconds to wait=u32 1000) -> ()  [unwired: 1 out]
          }
          frame #4 {
            n420 = case shown="True" "Active cal after cal?" {
              frame False {
              }
              frame True {
                n421 = local write "Active Cal"(TRUE ("Active Cal")) -> ()
                n422 = Wait (ms)(milliseconds to wait=u32 8000) -> ()  [unwired: 1 out]
              }
            }
          }
          frame #5 {
            n423 = property on="Save Calibration" class="Bool (strict)"("Val(Sgnl)"=TRUE ("Value (Signaling)")) -> ()  [unwired: 2 in, 2 out]
          }
          frame #6 {
            n424 = Wait (ms)(milliseconds to wait=u32 2000) -> ()  [unwired: 1 out]
          }
          frame #7 {
            # "Check to see if \nsaving done"
            n425 = while {
              stop <- w831 stop-if-true
              n426 = local read "Saving..."() -> (w832:bool)
              n427 = Wait (ms)(milliseconds to wait=u32 100) -> ()  [unwired: 1 out]
              n428 = Not(x=w832) -> (.not. x?=w831:bool)
            }
          }
          frame #8 {
            n429 = case shown="True" "W/ Offset 1" {
              tunnel: w835 -> [_ w836]
              frame False {
              }
              frame True {
                n430 = stacked-sequence {
                  tunnel: w836 -> [_ _ _ _ _ _ _ w853]
                  frame #0 {
                    n431 = property on="Trap Delta (MHz)" class="DigNum (strict)"("Val(Sgnl)"="Offset 1 Start (MHz)") -> ()  [unwired: 2 in, 2 out]
                    n432 = Replace Array Subset(array=u32[] [0] ("Index Values"), new element="Offset 1 Set", index=0) -> (w838:u32[])
                    n433 = property on="Saved AOD Raster Scan Parameter Sets" class="Arr (strict)"("Index Values"=w838) -> ()  [unwired: 2 in, 2 out]
                    n434 = property on="manual raster set" class="Ring (strict)"("Value"="Offset 1 Set") -> ()  [unwired: 2 in, 2 out]
                  }
                  frame #1 {
                    n435 = Wait (ms)(milliseconds to wait=u32 200) -> ()  [unwired: 1 out]
                  }
                  frame #2 {
                    n436 = property on="Load parameters" class="Bool (strict)"("Val(Sgnl)"=TRUE ("Value (Signaling)")) -> ()  [unwired: 2 in, 2 out]
                  }
                  frame #3 {
                    n437 = Wait (ms)(milliseconds to wait=u32 200) -> ()  [unwired: 1 out]
                  }
                  frame #4 {
                    n438 = property on="Trap Raster Scan" class="Bool (strict)"("Val(Sgnl)"=TRUE ("Value (Signaling)")) -> ()  [unwired: 2 in, 2 out]
                  }
                  frame #5 {
                    n439 = Wait (ms)(milliseconds to wait=u32 2000) -> ()  [unwired: 1 out]
                  }
                  frame #6 {
                    n440 = while {
                      stop <- w850 stop-if-true
                      n441 = local read "Raster Scanning..."() -> (w852:bool)
                      n442 = local read "Saving..."() -> (w848:bool)
                      n443 = Wait (ms)(milliseconds to wait=u32 100) -> ()  [unwired: 1 out]
                      n444 = Not(x=w848) -> (.not. x?=w847:bool)
                      n445 = Not(x=w852) -> (.not. x?=w849:bool)
                      n446 = And(x=w849, y=w847) -> (x .and. y?=w850:bool)
                    }
                  }
                  frame #7 {
                    n447 = property on="Trap Delta (MHz)" class="DigNum (strict)"("Val(Sgnl)"=w853) -> ()  [unwired: 2 in, 2 out]
                  }
                }
              }
            }
          }
          frame #9 {
            n448 = local read "Save ave N"() -> (w855:dbl)
            n449 = case shown="True" "W/ Offset 2" {
              tunnel: w856 -> [_ w863]
              tunnel: w855 -> [_ w862]
              tunnel: w854 -> [w858 _]
              frame False {
                n450 = case shown="False" w858 {
                  frame False {
                    n451 = Multiply(x="Cal read wait (s)", y=u32 1000 ("milliseconds to wait")) -> (x*y=w860:u32)
                    n452 = Wait (ms)(milliseconds to wait=w860) -> ()  [unwired: 1 out]
                  }
                  frame True {
                  }
                }
              }
              frame True {
                n453 = stacked-sequence {
                  tunnel: w863 -> [_ _ _ _ _ _ _ _ _ w884 _ _]
                  tunnel: w862 -> [_ _ _ _ _ _ _ _ _ w882 _ _]
                  frame #0 {
                    n454 = property on="Save ave N" class="DigNum (strict)"("Val(Sgnl)"=1.0 ("Value (Signaling)")) -> ()  [unwired: 2 in, 2 out]
                  }
                  frame #1 {
                    n455 = Wait (ms)(milliseconds to wait=u32 500) -> ()  [unwired: 1 out]
                  }
                  frame #2 {
                    n456 = property on="Trap Delta (MHz)" class="DigNum (strict)"("Val(Sgnl)"="Offset 2 Start (MHz)") -> ()  [unwired: 2 in, 2 out]
                    n457 = Replace Array Subset(array=u32[] [0] ("Index Values"), new element="Offset 2 Set", index=0) -> (w868:u32[])
                    n458 = property on="Saved AOD Raster Scan Parameter Sets" class="Arr (strict)"("Index Values"=w868) -> ()  [unwired: 2 in, 2 out]
                  }
                  frame #3 {
                    n459 = Wait (ms)(milliseconds to wait=u32 500) -> ()  [unwired: 1 out]
                  }
                  frame #4 {
                    n460 = property on="Load parameters" class="Bool (strict)"("Val(Sgnl)"=TRUE ("Value (Signaling)")) -> ()  [unwired: 2 in, 2 out]
                  }
                  frame #5 {
                    n461 = Wait (ms)(milliseconds to wait=u32 500) -> ()  [unwired: 1 out]
                  }
                  frame #6 {
                    n462 = property on="Trap Raster Scan" class="Bool (strict)"("Val(Sgnl)"=TRUE ("Value (Signaling)")) -> ()  [unwired: 2 in, 2 out]
                  }
                  frame #7 {
                    n463 = Wait (ms)(milliseconds to wait=u32 2000) -> ()  [unwired: 1 out]
                  }
                  frame #8 {
                    n464 = while {
                      stop <- w877 stop-if-true
                      n465 = local read "Raster Scanning..."() -> (w880:bool)
                      n466 = local read "Saving..."() -> (w878:bool)
                      n467 = Wait (ms)(milliseconds to wait=u32 100) -> ()  [unwired: 1 out]
                      n468 = Not(x=w878) -> (.not. x?=w876:bool)
                      n469 = Not(x=w880) -> (.not. x?=w879:bool)
                      n470 = And(x=w879, y=w876) -> (x .and. y?=w877:bool)
                    }
                  }
                  frame #9 {
                    n471 = property on="Trap Delta (MHz)" class="DigNum (strict)"("Val(Sgnl)"=w884) -> ()  [unwired: 2 in, 2 out]
                    n472 = property on="Saved AOD Raster Scan Parameter Sets" class="Arr (strict)"("Index Values"=u32[] [0]) -> ()  [unwired: 2 in, 2 out]
                    n473 = property on="Save ave N" class="DigNum (strict)"("Val(Sgnl)"=w882) -> ()  [unwired: 2 in, 2 out]
                  }
                  frame #10 {
                    n474 = Wait (ms)(milliseconds to wait=u32 500) -> ()  [unwired: 1 out]
                  }
                  frame #11 {
                    n475 = property on="Load parameters" class="Bool (strict)"("Val(Sgnl)"=TRUE ("Value (Signaling)")) -> ()  [unwired: 2 in, 2 out]
                  }
                }
              }
            }
          }
          frame #10 {
            # "Added by Ronen for flow calibration"
            n476 = case shown="True" "Flow based calibration?" {
              frame False {
              }
              frame True {
                n477 = stacked-sequence {
                  frame #0 {
                    n478 = local write "Flow Cal"(TRUE) -> ()
                  }
                  frame #1 {
                  }
                  frame #2 {
                    n479 = Wait (ms)(milliseconds to wait=u32 8000) -> ()  [unwired: 1 out]
                  }
                }
              }
            }
          }
          frame #11 {
            n480 = property on="Read Cal" class="Bool (strict)"("Val(Sgnl)"=TRUE ("Value (Signaling)")) -> ()  [unwired: 2 in, 2 out]
          }
          frame #12 {
            n481 = Wait (ms)(milliseconds to wait=u32 1000) -> ()  [unwired: 1 out]
          }
          frame #13 {
            n482 = property on="Fish for Tether" class="Bool (strict)"("Val(Sgnl)"="Fish after cal?") -> ()  [unwired: 2 in, 2 out]
          }
        }
        n483 = local write "Cal/Data Acq. Spot"(FALSE ("Cal/Data Acq. Spot")) -> ()
      }
      event "Dump Beads": Value Change {
        n484 = event-data() -> ()  [unwired: 1 in, 5 out]
        n485 = flat-sequence {
          tunnel: ["Dump spot flow on?"] -> w893
          tunnel: [w904] -> w894
          tunnel: w893 -> [w904]
          tunnel: w897 -> [w909]
          tunnel: w896 -> [w908]
          tunnel: [w906] -> w895
          tunnel: w894 -> [w906]
          tunnel: w895 -> [w919]
          frame #0 {
            w898 = FALSE ("Value (Signaling)")
            n486 = local read "Saving..."() -> (w900:bool)
            n487 = local write "Dump Beads"(FALSE ("Dump Beads")) -> ()
            n488 = property on="Inject Pump 3" class="Bool (strict)"("Val(Sgnl)"=w898) -> ()  [unwired: 2 in, 2 out]
            n489 = property on="Inject Pump 1" class="Bool (strict)"("Val(Sgnl)"=w898) -> ()  [unwired: 2 in, 2 out]
            n490 = local write "Stop Saving"(w900) -> ()
          }
          frame #1 {
            w901 = FALSE ("Fl. Triggered...")
            n491 = case shown="True" "Dump spot flow on?" {
              frame False {
              }
              frame True {
                n492 = property on="Sample Channel\nFlow" class="Bool (strict)"("Val(Sgnl)"=TRUE ("Stage Moving")) -> ()  [unwired: 2 in, 2 out]
              }
            }
            n493 = local write "Fl. Triggered..."(w901) -> ()
            n494 = local write "Tether"(w901) -> ()
